vi "peak_detection_testing.vi"() -> ()   [LabVIEW 2018]
doc: "Demonstrates the use of the Peak Detector VI."
uses:
  <vilib>/Utility/file.llb/Read Delimited Spreadsheet (DBL).vi
panel:
  out "Peaks Found":i32=9
  in  "threshold":dbl=1.0 format="%0.2f"
  in  "peak detector width":i32=1000 min=3
  in  "Filter Width":i32=100
  out "Uncorrected Thickness":dbl=0.19594166666649926
  in  "Length":i32=100
  in  "Size":i32=7830
  out "Execution Time":u32=930
  out "Signal Plot":cluster{"all rows":dbl[], "all rows":dbl[]}[](graph)
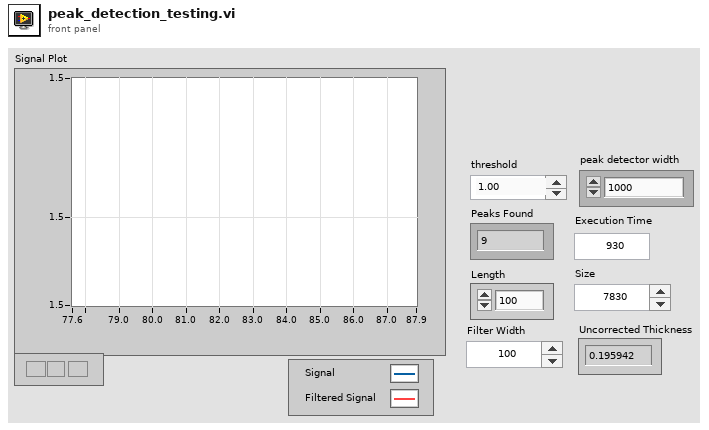
[diagram p1: front panel]
types:
  T1 = cluster{"Moving Averaged Array":dbl[], "Moving Averaged Array":dbl[]}
  T2 = cluster{"Block Averaged Array":dbl[], "Block Averaged Array":dbl[]}
  T3 = cluster{"Moving Averaged Array":dbl[], "Moving Averaged Array":dbl[]}[]
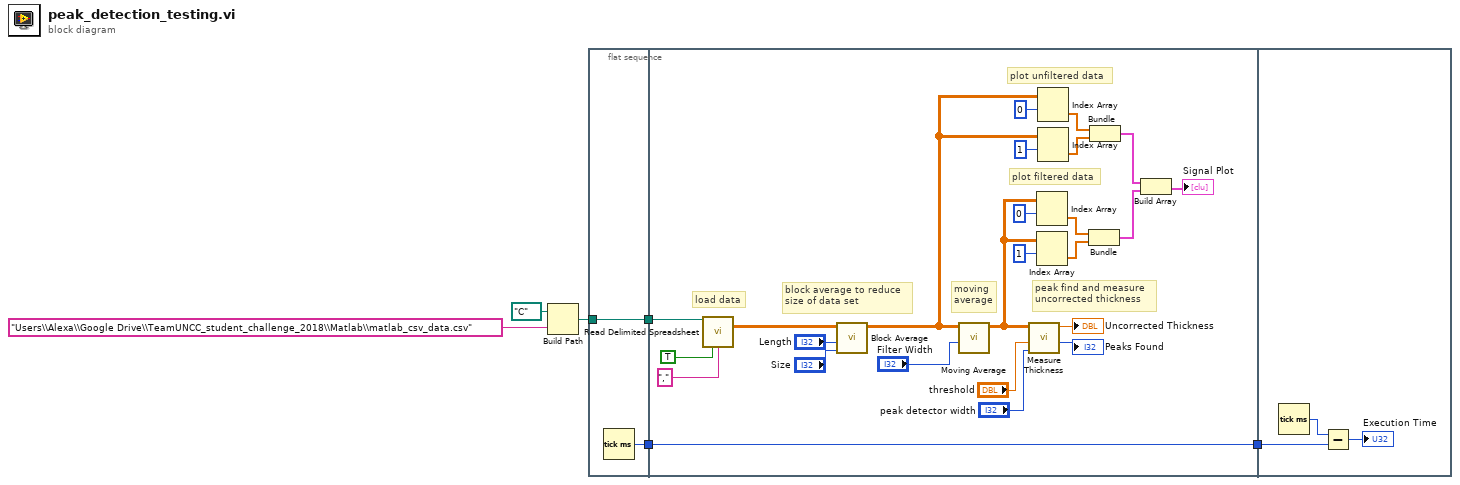
[diagram p0: block diagram]
diagram:
  n1 = Build Path(base path=path "C:/", name or relative path="Users\\Alexa\\Google Drive\\TeamUNCC_student_challenge_2018\\Matlab\\matlab_csv_data.csv") -> (appended path=w2:path)
  n2 = flat-sequence {
    tunnel: [w8] -> w6
    tunnel: w2 -> [w7]
    tunnel: [w7] -> w1
    tunnel: w6 -> [w31]
    tunnel: [w31] -> w5
    tunnel: w1 -> [w30]
    tunnel: w5 -> [w35]
    frame #0 {
      n3 = Tick Count (ms)() -> (millisecond timer value=w8:u32)
    }
    frame #1 {
      # "plot unfiltered data"
      # "plot filtered data"
      # "peak find and measure\nuncorrected thickness"
      # "moving\naverage"
      # "block average to reduce\nsize of data set"
      # "load data"
      n4 = call-poly <vilib>:"Read Delimited Spreadsheet.vi"("file path (dialog if empty)"=w30, "transpose? (F)"=TRUE, "delimiter (\\t)"=",") -> ("all rows"=w29:dbl[][])  [unwired: 7 in, 5 out]
      n5 = call "Block Average.vi"(8:"Size", "Subset Length"="Length", "Input Array"=w29) -> ("Block Averaged Array"=w10:dbl[][])  [unwired: 8 in]
      n6 = call "Moving Average.vi"("Filter Width"="Filter Width", "Input Array"=w10) -> ("Moving Averaged Array"=w19:dbl[][])  [unwired: 9 in]
      n7 = call "Measure Thickness.vi"("peak detector width"="peak detector width", "threshold"="threshold", "Input Array"=w19) -> ("peaks found"=→"Peaks Found":i32, "uncorrected thickness"=→"Uncorrected Thickness":dbl)  [unwired: 5 in, 2 out]
      n8 = Index Array(array=w19, index (row)=0) -> (element=w18:dbl[])  [unwired: 1 in]
      n9 = Index Array(array=w19, index (row)=1) -> (element=w17:dbl[])  [unwired: 1 in]
      n10 = Index Array(array=w10, index (row)=0) -> (element=w12:dbl[])  [unwired: 1 in]
      n11 = Index Array(array=w10, index (row)=1) -> (element=w11:dbl[])  [unwired: 1 in]
      n12 = Bundle("Moving Averaged Array"=w18, "Moving Averaged Array"=w17) -> (w16:T1)  [unwired: 1 in]
      n13 = Bundle("Block Averaged Array"=w12, "Block Averaged Array"=w11) -> (w9:T2)  [unwired: 1 in]
      n14 = Build Array(w9, w16) -> (→"Signal Plot":T3)
    }
    frame #2 {
      n15 = Tick Count (ms)() -> (millisecond timer value=w36:u32)
      n16 = Subtract(x=w36, y=w35) -> (x-y=→"Execution Time":u32)
    }
  }
